vi "initial arm.vi"   [LabVIEW 2018]
uses:
  ARM angles.vi
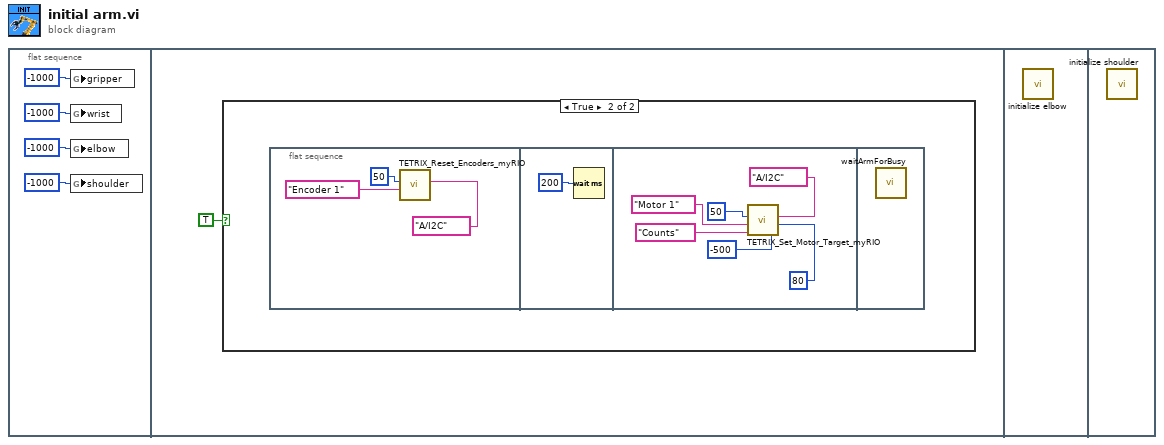
[diagram p0: block diagram]
diagram:
  n1 = flat-sequence {
    frame #0 {
      n2 = global write "ARM angles.vi" "gripper"(-1000 ("shoulder")) -> ()
      n3 = global write "ARM angles.vi" "wrist"(-1000 ("shoulder")) -> ()
      n4 = global write "ARM angles.vi" "elbow"(-1000 ("shoulder")) -> ()
      n5 = global write "ARM angles.vi" "shoulder"(-1000 ("shoulder")) -> ()
    }
    frame #1 {
      n6 = case shown="True" TRUE {
        frame False {
        }
        frame True {
          n7 = flat-sequence {
            frame #0 {
              n8 = call <vilib>:"TETRIX_Reset_Encoders_myRIO.vi"("myRIO MXP Port A/B"=tag "A/I2C", "Select Encoder"="Encoder 1", "Controller ID#  (I2C Address)"=u8 50) -> ()  [unwired: 4 in, 1 out]
            }
            frame #1 {
              n9 = Wait (ms)(milliseconds to wait=u32 200) -> ()  [unwired: 1 out]
            }
            frame #2 {
              n10 = call <vilib>:"TETRIX_Set_Motor_Target_myRIO.vi"("Motor Encoder Target"=-500, "Constant Speed (Degrees per Second)"=i16 80, "myRIO MXP Port A/B"=tag "A/I2C", "Encoder Units"="Counts", "Select Channel"="Motor 1", "Controller ID#  (I2C Address)"=u8 50) -> ()  [unwired: 1 in, 1 out]
            }
            frame #3 {
              n11 = call "waitArmForBusy.vi"() -> ()  [unwired: 12 in]
            }
          }
        }
      }
    }
    frame #2 {
      n12 = call "initialize elbow.vi"() -> ()  [unwired: 12 in]
    }
    frame #3 {
      n13 = call "initialize shoulder.vi"() -> ()  [unwired: 12 in]
    }
  }
